vi "19.MeasureDistance.vi"() -> ()   [LabVIEW 2017]
uses:
  <vilib>/userdefined/High Color/IMAQdx.ctl
  <vilib>/vision/driver/NI_Vision_Acquisition_Software.lvlib
  <vilib>/vision/NI_Vision_Development_Module.lvlib
panel:
  out "距离（单位：cm）":dbl
  out "Radius":i32
  out "Circles Data":T1(array[cluster])
  out "Image Out":T2(plugin-control)
  out "error out":errorcluster
  out "Image Hull":T2(plugin-control)
  out "Image Gaussian Filter":T2(plugin-control)
  out "Image Threshold":T2(plugin-control)
  in  "Camera Select":T3
  in  "停止":bool
  out "Image In":T2(plugin-control)
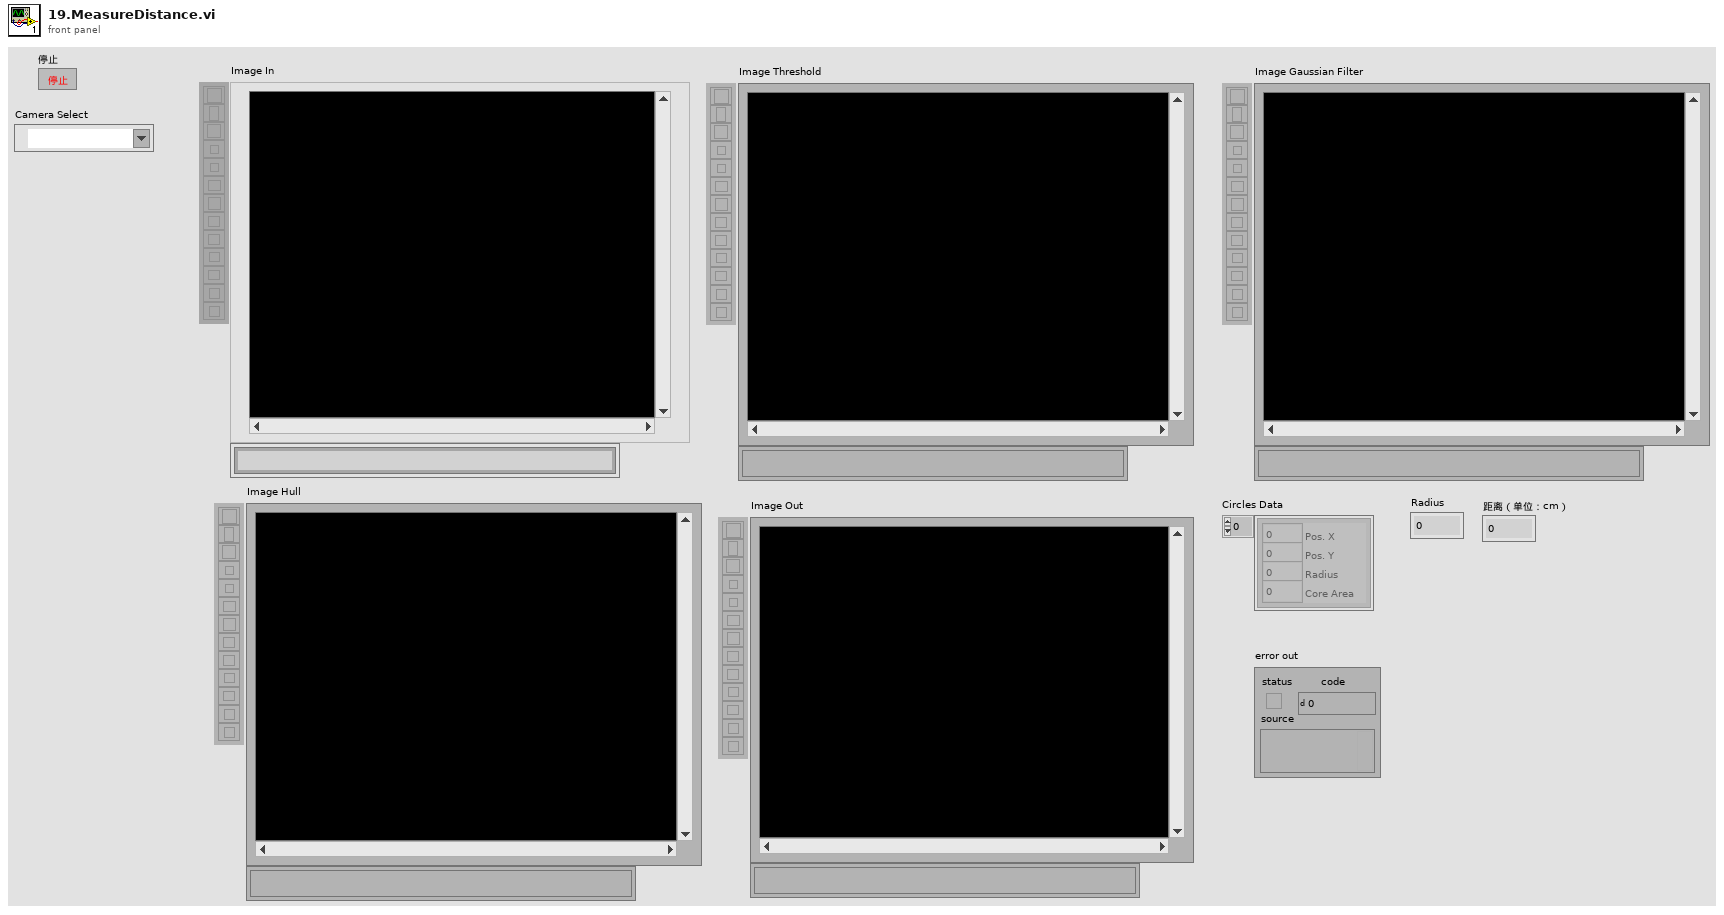
[diagram p1: front panel]
types:
  T1 = cluster{"Pos. X":i32, "Pos. Y":i32, "Radius":i32, "Core Area":i32}[]
  T2 = typedef "IMAQ Image.ctl" = refnum<image>
  T3 = typedef "IMAQdx.ctl" = refnum<k21>
  T4 = cluster{"Pos. X":i32, "Pos. Y":i32, "Radius":i32, "Core Area":i32}
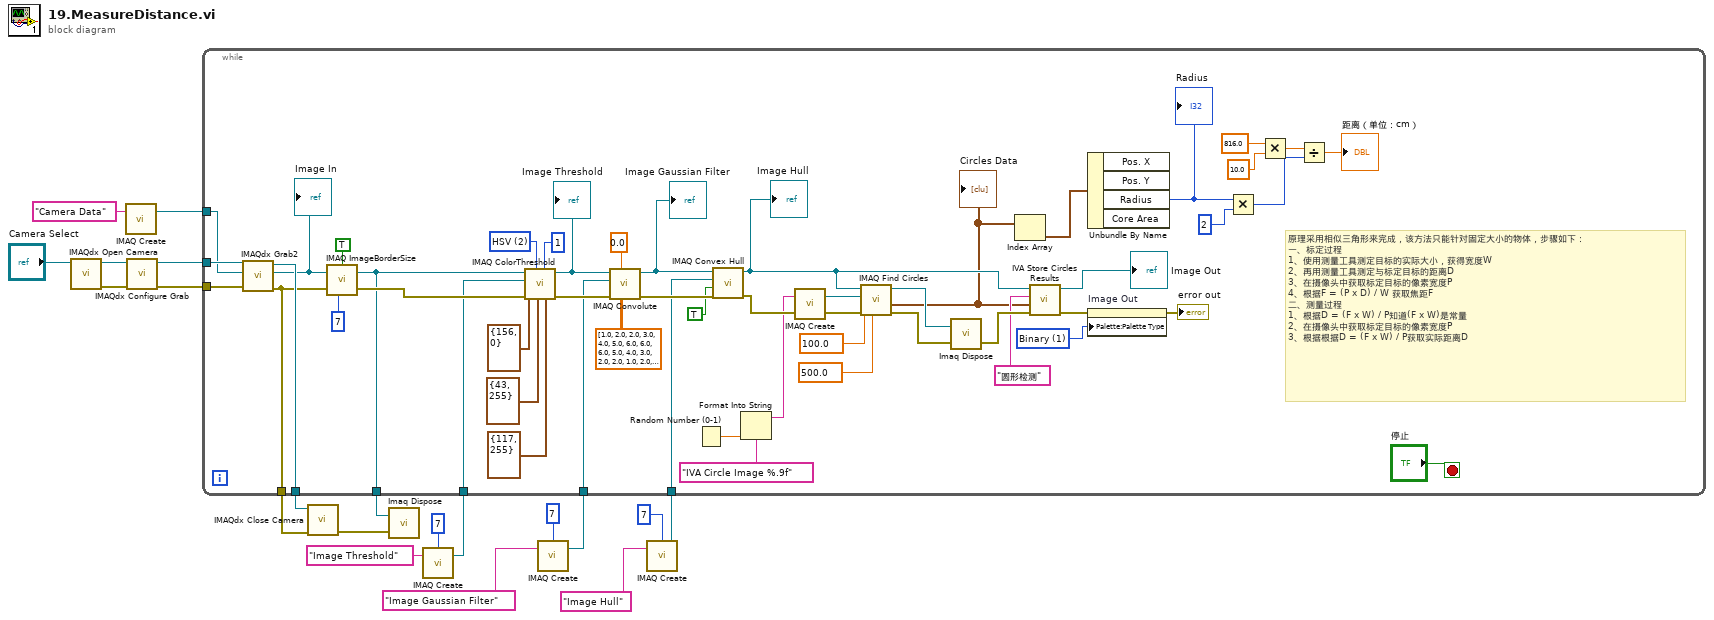
[diagram p0: block diagram]
diagram:
  n1 = call <vilib>:"IMAQdx Open Camera.vi"("Session In"="Camera Select") -> ("error out"=w20:errorcluster, "Session Out"=w19:T3)  [unwired: 9 in]
  n2 = call "IMAQ Create"("Image Name"="Camera Data") -> ("New Image"=w16:T2)  [unwired: 4 in, 1 out]
  n3 = call <vilib>:"IMAQdx Configure Grab.vi"("error in"=w20, "Session In"=w19) -> ("error out"=w17:errorcluster, "Session Out"=w18:T3)  [unwired: 8 in]
  n4 = call "IMAQ Create"("Border Size"=7, "Image Name"="Image Threshold") -> ("New Image"=w10:T2)  [unwired: 3 in, 1 out]
  n5 = call "IMAQ Create"("Border Size"=7, "Image Name"="Image Gaussian Filter") -> ("New Image"=w6:T2)  [unwired: 3 in, 1 out]
  n6 = call "IMAQ Create"("Border Size"=7, "Image Name"="Image Hull") -> ("New Image"=w3:T2)  [unwired: 3 in, 1 out]
  n7 = while {
    tunnel: w18 -> [w72]
    tunnel: w17 -> [w71]
    tunnel: w16 -> [w70]
    tunnel: [w60] -> w14
    tunnel: [w59] -> w13
    tunnel: [w58] -> w11
    tunnel: w10 -> [w56]
    tunnel: w6 -> [w53]
    tunnel: w3 -> [w48]
    stop <- "停止" stop-if-true
    w36 = u32 1 items=["Grayscale", "Binary", "Gradient", "Rainbow", "Temperature", "User Defined", "Binary 16 Bit", "Gradient 16 Bit", "Rainbow 16 Bit", "Temperature 16 Bit", "User Defined 16 Bit"] ("Palette Type")
    w66 = u16 2 items=["RGB", "HSL", "HSV", "HSI"] ("Color Mode")
    # "原理采用相似三角形来完成，该方法只能针对固定大小的物体，步骤如下：\n一、标定过程\n1、使用测量工具测定目标的实际大小，获得宽度W\n2、再用测量工具测定与标定目标的距离D\n3、在摄像头中获取标定目标的像素宽度P\n4、根据F = (P x D) / W 获取焦距F\n二、测量过程\n1、根据D = (F x W) / P知道(F x W)是常量\n2、在摄像头中获取标定目标的像素宽度P\n3、根据根据D = (F x W) / P获取实际距离D"
    n8 = call <vilib>:"IMAQdx Grab2.vi"("error in"=w71, "Image In"=w70, "Session In"=w72) -> ("error out"=w59:errorcluster, "Image Out"=w57:T2, "Session Out"=w60:T3)  [unwired: 5 in, 1 out]
    "Image In" <- w57
    n9 = call "IMAQ ImageBorderSize"("Get/Set Status? (Set)"=TRUE, "Image"=w57, "Image border size in"=7, "error in (no error)"=w59) -> ("Image Out"=w58:T2, "error out"=w67:errorcluster)  [unwired: 1 out]
    n10 = call "IMAQ ColorThreshold"("Blue or Luma or Val or Inten Range"=cluster{"Lower value":i32, "Upper value":i32} {"Lower value"=117, "Upper value"=255}, "Replace Value"=1, "Green or Sat Range"=cluster{"Lower value":i32, "Upper value":i32} {"Lower value"=43, "Upper value"=255}, "Color Mode"=w66, "error in (no error)"=w67, "Red or Hue Range"=cluster{"Lower value":i32, "Upper value":i32} {"Lower value"=156, "Upper value"=0}, "Image Dst"=w56, "Image Src"=w58) -> ("error out"=w54:errorcluster, "Image Dst Out"=w55:T2)  [unwired: 2 out]
    "Image Threshold" <- w55
    n11 = call "IMAQ Convolute"("Kernel"=sgl[][] [[1.0, 2.0, 2.0, 3.0, 4.0, 5.0, 6.0, 6.0, 6.0, 5.0, 4.0, 3.0, 2.0, 2.0, 1.0], [2.0, 3.0, 4.0, 5.0, 7.0, 8.0, 9.0, 9.0, 9.0, 8.0, 7.0, 5.0, 4.0, 3.0, 2.0], [2.0, 4.0, 6.0, 8.0, 10.0, 12.0, 13.0, 13.0, 13.0, 12.0, 10.0, 8.0, 6.0, 4.0, 2.0], [3.0, 5.0, 8.0, 10.0, 13.0, 16.0, 18.0, 18.0, 18.0, 16.0, 13.0, 10.0, 8.0, 5.0, 3.0], [4.0, 7.0, 10.0, 13.0, 17.0, 21.0, 23.0, 24.0, 23.0, 21.0, 17.0, 13.0, 10.0, 7.0, 4.0], [5.0, 8.0, 12.0, 16.0, 21.0, 25.0, 27.0, 28.0, 27.0, 25.0, 21.0, 16.0, 12.0, 8.0, 5.0], [6.0, 9.0, 13.0, 18.0, 23.0, 27.0, 30.0, 31.0, 30.0, 27.0, 23.0, 18.0, 13.0, 9.0, 6.0], [6.0, 9.0, 13.0, 18.0, 24.0, 28.0, 31.0, 33.0, 31.0, 28.0, 24.0, 18.0, 13.0, 9.0, 6.0], [6.0, 9.0, 13.0, 18.0, 23.0, 27.0, 30.0, 31.0, 30.0, 27.0, 23.0, 18.0, 13.0, 9.0, 6.0], [5.0, 8.0, 12.0, 16.0, 21.0, 25.0, 27.0, 28.0, 27.0, 25.0, 21.0, 16.0, 12.0, 8.0, 5.0], [4.0, 7.0, 10.0, 13.0, 17.0, 21.0, 23.0, 24.0, 23.0, 21.0, 17.0, 13.0, 10.0, 7.0, 4.0], [3.0, 5.0, 8.0, 10.0, 13.0, 16.0, 18.0, 18.0, 18.0, 16.0, 13.0, 10.0, 8.0, 5.0, 3.0], [2.0, 4.0, 6.0, 8.0, 10.0, 12.0, 13.0, 13.0, 13.0, 12.0, 10.0, 8.0, 6.0, 4.0, 2.0], [2.0, 3.0, 4.0, 5.0, 7.0, 8.0, 9.0, 9.0, 9.0, 8.0, 7.0, 5.0, 4.0, 3.0, 2.0], [1.0, 2.0, 2.0, 3.0, 4.0, 5.0, 6.0, 6.0, 6.0, 5.0, 4.0, 3.0, 2.0, 2.0, 1.0]], "Divider (kernel sum)"=sgl 0.0, "error in (no error)"=w54, "Image Mask"=w53, "Image Src"=w55) -> ("error out"=w50:errorcluster, "Image Dst Out"=w47:T2)  [unwired: 2 in, 3 out]
    "Image Gaussian Filter" <- w47
    n12 = Random Number (0-1)() -> (number: 0 to 1=w32:dbl)
    n13 = call "IMAQ Convex Hull"("error in (no error)"=w50, "Connectivity 4/8 (8)"=TRUE, "Image Dst"=w48, "Image Src"=w47) -> ("error out"=w34:errorcluster, "Image Dst Out"=w35:T2)  [unwired: 6 out]
    "Image Hull" <- w35
    n14 = Format Into String(format string="IVA Circle Image %.9f" ("Image Name"), w32) -> (resulting string=w31:string)  [unwired: 2 in, 1 out]
    n15 = call "IMAQ Create"("Image Name"=w31, "error in (no error)"=w34) -> ("New Image"=w44:T2, "error out"=w43:errorcluster)  [unwired: 2 in, 1 out]
    n16 = call "IMAQ Find Circles"("Max Radius"=sgl 500.0, "error in (no error)"=w43, "Min Radius"=sgl 100.0, "Image Dst"=w44, "Image Src"=w35) -> ("error out"=w42:errorcluster, "Circles Data"=w29:T1, "Image Dst Out"=w30:T2)  [unwired: 4 out]
    "Circles Data" <- w29
    n17 = call "Imaq Dispose"("Image"=w30, "error in (no error)"=w42) -> ("error out"=w41:errorcluster)  [unwired: 1 in, 3 out]
    n18 = Index Array(array=w29) -> (element=w28:T4)  [unwired: 1 in]
    n19 = call <vilib>:"IVA Store Circles Results.vi"("error in (no error)"=w41, "Circles Data"=w29, "Step Name"="圆形检测", "Image in"=w35) -> ("error out"=w39:errorcluster, "Image dup"=→"Image Out":T2)  [unwired: 6 out]
    n20 = Unbundle By Name(w28) -> ("Radius"=w27:i32)  [unwired: 3 out]
    "Radius" <- w27
    n21 = property on="Image Out" class="ImageControl"(error in=w39, "Palette:Palette Type"=w36) -> (error out=→"error out":errorcluster)  [unwired: 1 in, 1 out]
    n22 = Multiply(x=w27, y=2) -> (x*y=w22:i32)
    n23 = Multiply(x=816.0, y=10.0) -> (x*y=w23:dbl)
    n24 = Divide(x=w23, y=w22) -> (x/y=→"距离（单位：cm）":dbl)
  }
  n25 = call <vilib>:"IMAQdx Close Camera.vi"("error in"=w13, "Session In"=w14) -> ("error out"=w12:errorcluster)  [unwired: 9 in]
  n26 = call "Imaq Dispose"("Image"=w11, "error in (no error)"=w12) -> ()  [unwired: 4 in, 1 out]
